vi "Generator DC Sweep Manager_old.vi"(8 "error in (no error)":errorcluster, 10 "sweep index":i32=-1, 11 "Lockin.DAQ in":refnum<class "Lockin.DAQ.lvclass">) -> (0 "error out":errorcluster, 1 "Start (V)":dbl[](array[numeric]), 2 "End (V)":dbl[](array[numeric]), 3 "Lockin.DAQ out":refnum<class "Lockin.DAQ.lvclass">)   [LabVIEW 2016, in "Lockin.DAQ.lvclass"]
uses:
  Lockin.DAQ.lvclass
  Lockin.DAQ.lvclass/Lockin.DAQ.ctl
panel:
  out "ms":u32
  out "time":dbl
  out "sweeping":dbl
  out "start sweep time":timestamp
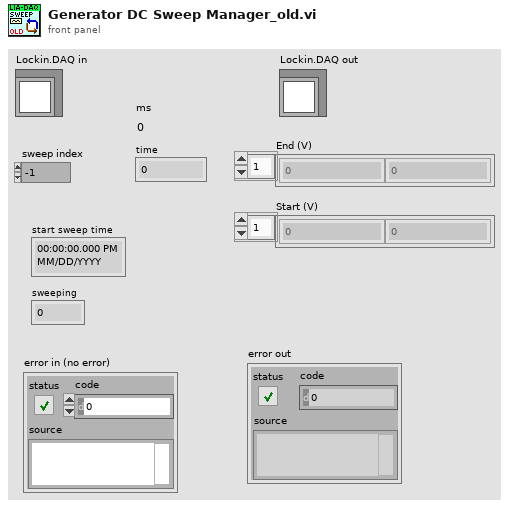
[diagram p1: front panel]
types:
  T1 = typedef "Lockin.DAQ.lvclass/AO-cluster.ctl" = cluster{"Ch":i32[], "Amp (V)":dbl[], "DC (V)":dbl[], "f (Hz)":dbl[], "Phase (°)":dbl[], "Function":T2[], "Sweep?":bool[]}
  T2 = typedef "Lockin.DAQ.lvclass/Function-enum.ctl" = enum16{"Sine", "Triangle", "Square", "Sawtooth"}
  T3 = typedef "Lockin.DAQ.lvclass/Sweep Configuration--Cluster.ctl" = cluster{"Sweep Time (s)":dbl, "Initial Wait (s)":dbl, "Sweep Channel":i32[], "Sweep Start (V)":dbl[], "Sweep End (V)":dbl[], "Pattern":T4[], "Return to Start":bool}
  T4 = typedef "Lockin.DAQ.lvclass/Sweep Pattern--Enum.ctl" = enum16{"Ramp /", "Ramp /\\", "Smooth Ramp _/", "Smooth Ramp _/\\_", "Frequency"}
  T5 = typedef "Lockin.DAQ.lvclass/Sampling.ctl" = cluster{"Fs":dbl, "#s":i32}
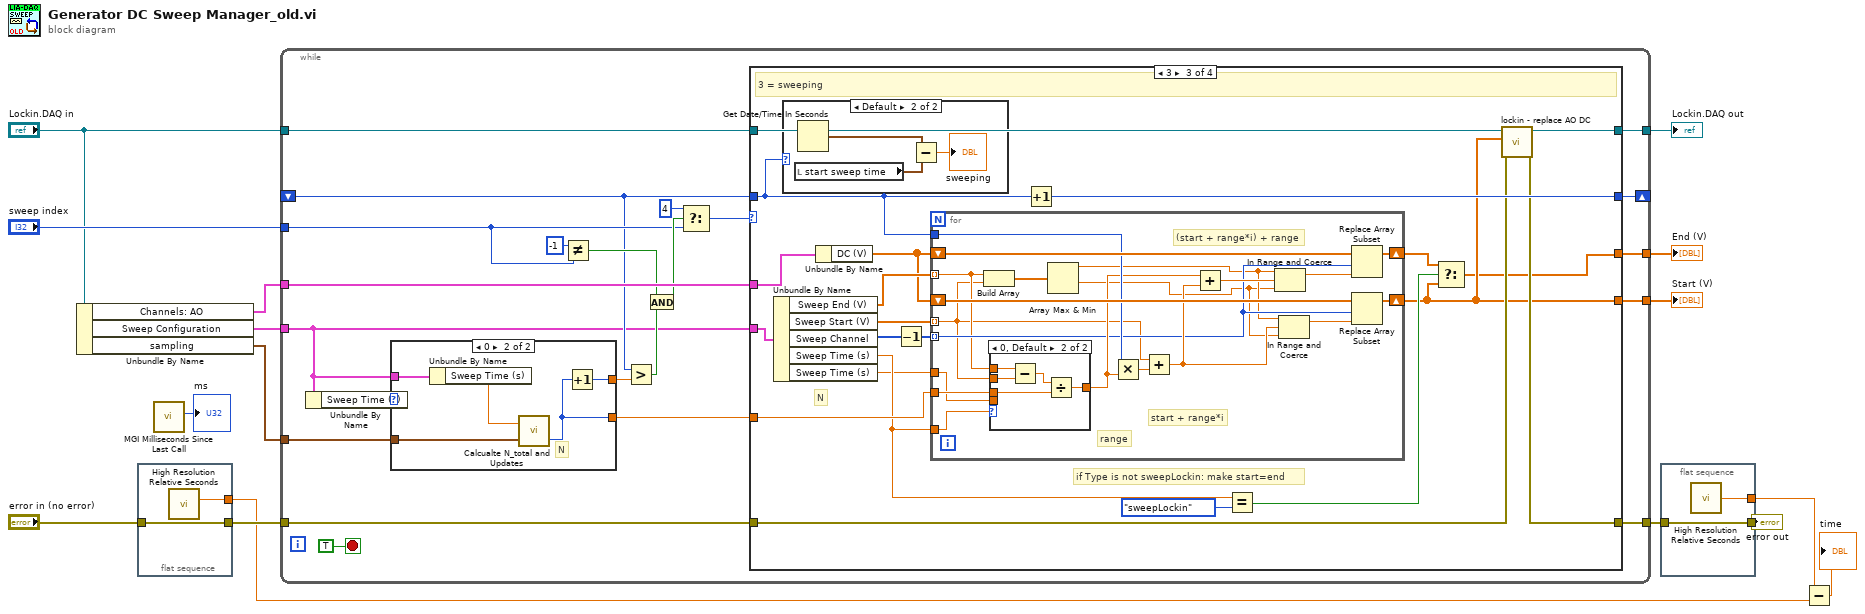
[diagram p0: block diagram]
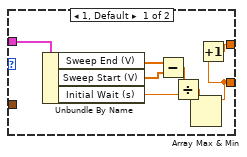
[diagram p2: hidden frame]
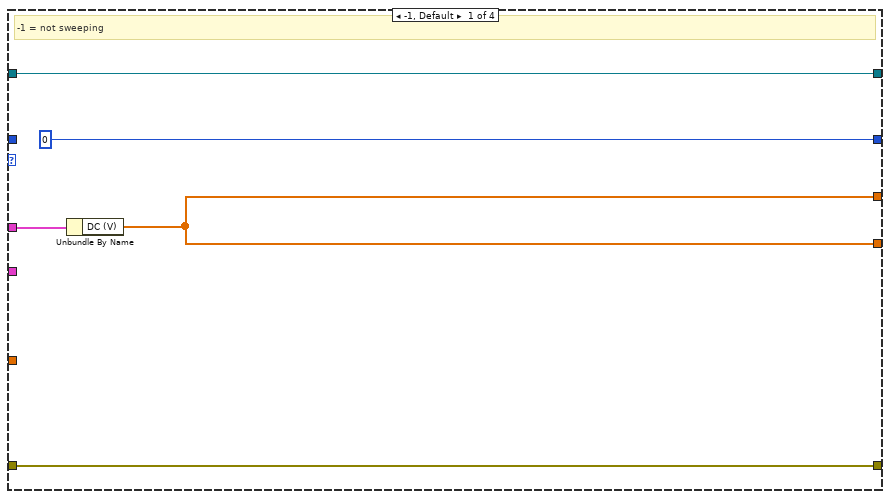
[diagram p3: hidden frame]
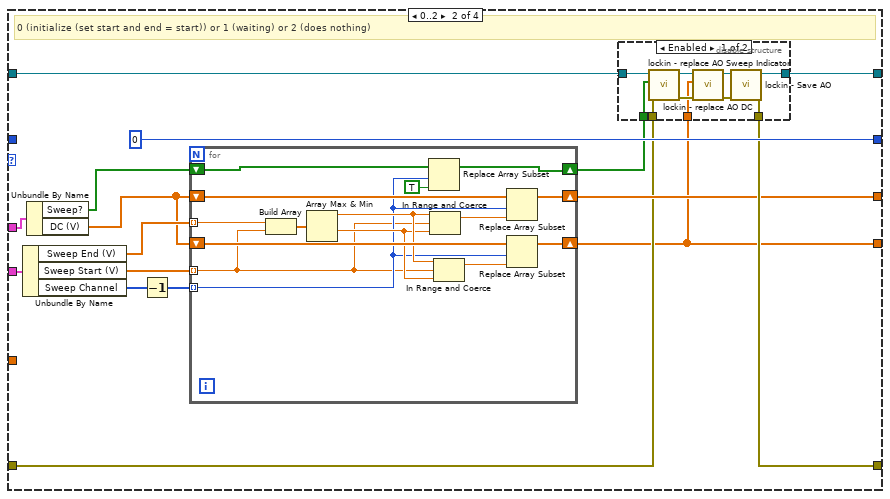
[diagram p4: hidden frame]
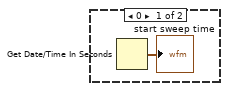
[diagram p6: hidden frame]
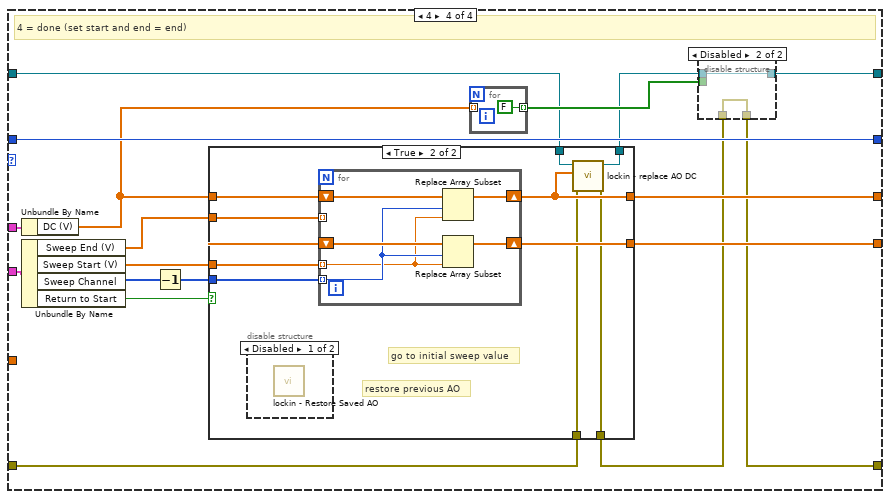
[diagram p8: hidden frame]
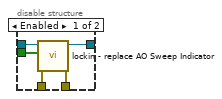
[diagram p9: hidden frame]
diagram:
  n1 = Unbundle By Name("Lockin.DAQ in") -> ("Channels: AO"=w12:T1, "Sweep Configuration"=w13:T3, "sampling"=w14:T5)
  n2 = flat-sequence {
    tunnel: "error in (no error)" -> [w18]
    tunnel: [w18] -> w7
    tunnel: [w17] -> w3
    frame #0 {
      n3 = call <vilib>:"High Resolution Relative Seconds.vi"() -> ("relative seconds"=w17:dbl)
    }
  }
  n4 = call <userlib>:"MGI Milliseconds Since Last Call.vi"() -> ("ms"=→"ms":u32)  [unwired: 6 in, 1 out]
  n5 = while {
    tunnel: w12 -> [w40]
    tunnel: [w25] -> w15
    tunnel: [w39] -> w16
    tunnel: w13 -> [w19]
    tunnel: "sweep index" -> [w24]
    tunnel: w14 -> [w36]
    shift-right: [w38] -> _
    shift-left: _ -> [w21]
    tunnel: [w29] -> w10
    tunnel: "Lockin.DAQ in" -> [w28]
    tunnel: w7 -> [w27]
    tunnel: [w26] -> w5
    stop <- TRUE stop-if-true
    n6 = Unbundle By Name(w19) -> ("Sweep Time (s)"=w23:dbl)
    n7 = case shown="0" w23 {
      tunnel: w36 -> [_ w49]
      tunnel: [w43 w51] -> w33
      tunnel: w19 -> [w41 w53]
      tunnel: [w42 w52] -> w22
      frame 1, Default {
        n8 = Unbundle By Name(w41) -> ("Sweep End (V)"=w48:dbl[], "Sweep Start (V)"=w47:dbl[], "Initial Wait (s)"=w45:dbl)
        n9 = Subtract(x=w48, y=w47) -> (x-y=w46:dbl[])
        n10 = Divide(x=w46, y=w45) -> (x/y=w44:dbl[])
        n11 = Array Max & Min(array=w44) -> (max value=w43:dbl)  [unwired: 3 out]
        n12 = Increment(x=w43) -> (x+1=w42:dbl)
      }
      frame 0 {
        # "N"
        n13 = Unbundle By Name(w53) -> ("Sweep Time (s)"=w50:dbl)
        n14 = call "Calcualte N_total and Updates.vi"("Sampling"=w49, "Sweep Time (s)"=w50) -> ("Updates"=w51:i32)  [unwired: 1 out]
        n15 = Increment(x=w51) -> (x+1=w52:i32)
      }
    }
    n16 = Not Equal?(x=-1, y=w24) -> (x != y?=w30:bool)
    n17 = Greater?(x=w21, y=w22) -> (0:w20:bool)
    n18 = And(x=w30, y=w20) -> (x .and. y?=w31:bool)
    n19 = Select(t=4, s=w31, f=w24) -> (s? t:f=w34:i32)
    n20 = case shown="3" w34 {
      tunnel: w40 -> [w58 w74 w122 w170]
      tunnel: [w57 w59 w104 w168] -> w39
      tunnel: w19 -> [_ w70 w118 w165]
      tunnel: [0 0 w115 w163] -> w38
      tunnel: w21 -> [_ _ w102 w163]
      tunnel: w33 -> [_ _ w114 _]
      tunnel: [w55 w66 w105 w154] -> w29
      tunnel: w28 -> [w55 w63 w112 w158]
      tunnel: w27 -> [w54 w61 w113 w156]
      tunnel: [w54 w65 w111 w153] -> w26
      tunnel: [w57 w64 w103 w162] -> w25
      frame -1, Default {
        # "-1 = not sweeping"
        n21 = Unbundle By Name(w58) -> ("DC (V)"=w57:dbl[])
      }
      frame 0..2 {
        # "0 (initialize (set start and end = start)) or 1 (waiting) or 2 (does nothing)"
        n22 = Unbundle By Name(w70) -> ("Sweep End (V)"=w71:dbl[], "Sweep Start (V)"=w72:dbl[], "Sweep Channel"=w73:i32[])
        n23 = Unbundle By Name(w74) -> ("Sweep?"=w62:bool[], "DC (V)"=w68:dbl[])
        n24 = Decrement(x=w73) -> (x-1=w69:i32[])
        n25 = for {
          shift-right: [w100] -> w64
          shift-left: w68 -> [w101]
          shift-right: [w98] -> w59
          shift-left: w68 -> [w99]
          tunnel: w72 -> [w87] mode=indexing
          tunnel: w71 -> [w94] mode=indexing
          tunnel: w69 -> [w89] mode=indexing
          shift-right: [w90] -> w60
          shift-left: w62 -> [w91]
          n26 = Build Array(w94, w87) -> (w95:dbl[])
          n27 = Array Max & Min(array=w95) -> (max value=w93:dbl, min value=w92:dbl)  [unwired: 2 out]
          n28 = Replace Array Subset(array=w91, new element=TRUE ("new element/subarray"), index=w89) -> (w90:bool[])
          n29 = In Range and Coerce(upper limit=w93, x=w87, lower limit=w92) -> (coerced(x)=w97:dbl)  [unwired: 1 out]
          n30 = In Range and Coerce(upper limit=w93, x=w87, lower limit=w92) -> (coerced(x)=w96:dbl)  [unwired: 1 out]
          n31 = Replace Array Subset(array=w101, new element=w97, index=w89) -> (w100:dbl[])
          n32 = Replace Array Subset(array=w99, new element=w96, index=w89) -> (w98:dbl[])
        }
        n33 = disable-structure shown="Enabled" {
          disable-tunnel: [w84 w86] -> w66
          disable-tunnel: [w83 w85] -> w65
          disable-tunnel: w63 -> [w81 w86]
          disable-tunnel: w61 -> [w78 w85]
          disable-tunnel: w60 -> [w76 _]
          disable-tunnel: w59 -> [w75 _]
          frame Enabled {
            n34 = call "lockin - replace AO Sweep Indicator.vi"("error in (no error)"=w78, "Channels: AO.Sweep?"=w76, "Lockin.DAQ"=w81) -> ("error out"=w79:errorcluster, "Lockin.DAQ out"=w80:refnum<class "Lockin.DAQ.lvclass">)  [unwired: 7 in]
            n35 = call "lockin - replace AO DC.vi"("error in (no error)"=w79, "AO.DC (V)"=w75, "LockinDAQ"=w80) -> ("error out"=w77:errorcluster, "LockinDAQ out"=w82:refnum<class "Lockin.DAQ.lvclass">)  [unwired: 7 in]
            n36 = call "lockin - Save AO.vi"("error in (no error)"=w77, "LockinDAQ"=w82) -> ("error out"=w83:errorcluster, "LockinDAQ out"=w84:refnum<class "Lockin.DAQ.lvclass">)  [unwired: 8 in]
          }
          frame Disabled {
          }
        }
      }
      frame 3 {
        # "if Type is not sweepLockin: make start=end"
        # "N"
        # "3 = sweeping"
        n37 = Unbundle By Name(w118) -> ("Sweep End (V)"=w119:dbl[], "Sweep Start (V)"=w120:dbl[], "Sweep Channel"=w121:i32[], "Sweep Time (s)"=w107:dbl, "Sweep Time (s)"=w106:dbl)
        n38 = case shown="Default" w102 {
          frame 0 {
            n39 = Get Date/Time In Seconds() -> (seconds since 1Jan1904=→"start sweep time":timestamp)
          }
          frame Default {
            n40 = local read "start sweep time"() -> (w125:timestamp)
            n41 = Get Date/Time In Seconds() -> (seconds since 1Jan1904=w124:timestamp)
            n42 = Subtract(x=w124, y=w125) -> (x-y=→"sweeping":dbl)
          }
        }
        n43 = Unbundle By Name(w122) -> ("DC (V)"=w116:dbl[])
        n44 = Decrement(x=w121) -> (x-1=w117:i32[])
        n45 = for {
          shift-right: [w145] -> w108
          shift-left: w116 -> [w146]
          shift-right: [w143] -> w104
          shift-left: w116 -> [w144]
          tunnel: w120 -> [w132] mode=indexing
          tunnel: w119 -> [w133] mode=indexing
          tunnel: w117 -> [w134] mode=indexing
          tunnel: w102 -> [w140]
          tunnel: w114 -> [w142]
          tunnel: w107 -> [w128]
          tunnel: w106 -> [w127]
          # "(start + range*i) + range"
          # "start + range*i"
          # "range"
          n46 = Build Array(w133, w132) -> (w131:dbl[])
          n47 = case shown="0, Default" w128 {
            tunnel: w142 -> [_ w152]
            tunnel: [w147 w150] -> w139
            tunnel: w133 -> [_ w149]
            tunnel: w132 -> [_ w148]
            tunnel: w127 -> [w147 _]
            frame 1 {
            }
            frame 0, Default {
              n48 = Subtract(x=w149, y=w148) -> (x-y=w151:dbl)
              n49 = Divide(x=w151, y=w152) -> (x/y=w150:dbl)
            }
          }
          n50 = Array Max & Min(array=w131) -> (max value=w130:dbl, min value=w129:dbl)  [unwired: 2 out]
          n51 = Multiply(x=w140, y=w139) -> (x*y=w141:dbl)
          n52 = Add(x=w132, y=w141) -> (x+y=w135:dbl)
          n53 = Add(x=w139, y=w135) -> (x+y=w138:dbl)
          n54 = In Range and Coerce(upper limit=w130, x=w138, lower limit=w129) -> (coerced(x)=w137:dbl)  [unwired: 1 out]
          n55 = In Range and Coerce(upper limit=w130, x=w135, lower limit=w129) -> (coerced(x)=w136:dbl)  [unwired: 1 out]
          n56 = Replace Array Subset(array=w146, new element=w137, index=w134) -> (w145:dbl[])
          n57 = Replace Array Subset(array=w144, new element=w136, index=w134) -> (w143:dbl[])
        }
        n58 = Increment(x=w102) -> (x+1=w115:i32)
        n59 = Equal?(x=w107, y=enum16{"sweepLockin", "sweepIV"}."sweepLockin" ("Type")) -> (x = y?=w109:bool)
        n60 = Select(t=w108, s=w109, f=w104) -> (s? t:f=w103:dbl[])
        n61 = call "lockin - replace AO DC.vi"("error in (no error)"=w113, "AO.DC (V)"=w104, "LockinDAQ"=w112) -> ("error out"=w111:errorcluster, "LockinDAQ out"=w105:refnum<class "Lockin.DAQ.lvclass">)  [unwired: 7 in]
      }
      frame 4 {
        # "4 = done (set start and end = end)"
        n62 = Unbundle By Name(w170) -> ("DC (V)"=w160:dbl[])
        n63 = Unbundle By Name(w165) -> ("Sweep End (V)"=w166:dbl[], "Sweep Start (V)"=w167:dbl[], "Sweep Channel"=w169:i32[], "Return to Start"=w161:bool)
        n64 = Decrement(x=w169) -> (x-1=w164:i32[])
        n65 = case shown="True" w161 {
          tunnel: [w181 w191] -> w168
          tunnel: w167 -> [_ w190]
          tunnel: w166 -> [_ w189]
          tunnel: w164 -> [_ w188]
          tunnel: w160 -> [w181 w187]
          tunnel: [w181 w184] -> w162
          tunnel: w158 -> [w180 w186]
          tunnel: [w180 w185] -> w157
          tunnel: w156 -> [w179 w183]
          tunnel: [w179 w182] -> w155
          frame False {
            # "remain at current value of DC"
          }
          frame True {
            # "restore previous AO"
            # "go to initial sweep value"
            n66 = disable-structure shown="Disabled" {
              frame Disabled {
                n67 = call "lockin - Restore Saved AO.vi"() -> ()  [unwired: 10 in, 2 out]
              }
              frame Enabled {
              }
            }
            n68 = for {
              shift-right: [w196] -> w184
              shift-left: w187 -> [w197]
              shift-right: [w194] -> w191
              shift-left: w187 -> [w195]
              tunnel: w190 -> [w192] mode=indexing
              tunnel: w189 -> [_] mode=indexing
              tunnel: w188 -> [w193] mode=indexing
              n69 = Replace Array Subset(array=w197, new element=w192, index=w193) -> (w196:dbl[])
              n70 = Replace Array Subset(array=w195, new element=w192, index=w193) -> (w194:dbl[])
            }
            n71 = call "lockin - replace AO DC.vi"("error in (no error)"=w183, "AO.DC (V)"=w184, "LockinDAQ"=w186) -> ("error out"=w182:errorcluster, "LockinDAQ out"=w185:refnum<class "Lockin.DAQ.lvclass">)  [unwired: 7 in]
          }
        }
        n72 = for {
          tunnel: w160 -> [_] mode=indexing
          tunnel: [FALSE] -> w159 mode=indexing
        }
        n73 = disable-structure shown="Disabled" {
          disable-tunnel: w159 -> [w175 _]
          disable-tunnel: w157 -> [w174 w177]
          disable-tunnel: w155 -> [w173 w176]
          disable-tunnel: [w172 w177] -> w154
          disable-tunnel: [w171 w176] -> w153
          frame Enabled {
            n74 = call "lockin - replace AO Sweep Indicator.vi"("error in (no error)"=w173, "Channels: AO.Sweep?"=w175, "Lockin.DAQ"=w174) -> ("error out"=w171:errorcluster, "Lockin.DAQ out"=w172:refnum<class "Lockin.DAQ.lvclass">)  [unwired: 7 in]
          }
          frame Disabled {
          }
        }
      }
    }
  }
  "Start (V)" <- w16
  "End (V)" <- w15
  "Lockin.DAQ out" <- w10
  n75 = flat-sequence {
    tunnel: w5 -> [w199]
    tunnel: [w199] -> w6
    tunnel: [w198] -> w4
    frame #0 {
      n76 = call <vilib>:"High Resolution Relative Seconds.vi"() -> ("relative seconds"=w198:dbl)
    }
  }
  n77 = Subtract(x=w4, y=w3) -> (x-y=→"time":dbl)
  "error out" <- w6
